vi "Read Description map.vi"(8 "error in (no error)":errorcluster, 11 "Test Tree in":refnum<class "Test Tree.lvclass">) -> (0 "error out":errorcluster, 2 "Description map":map{string, string}(c390), 3 "Test Tree out":refnum<class "Test Tree.lvclass">)   [LabVIEW 2020, in "Test Tree.lvclass"]
uses:
  Test Tree.lvclass
  Test Tree.lvclass/Test Tree.ctl
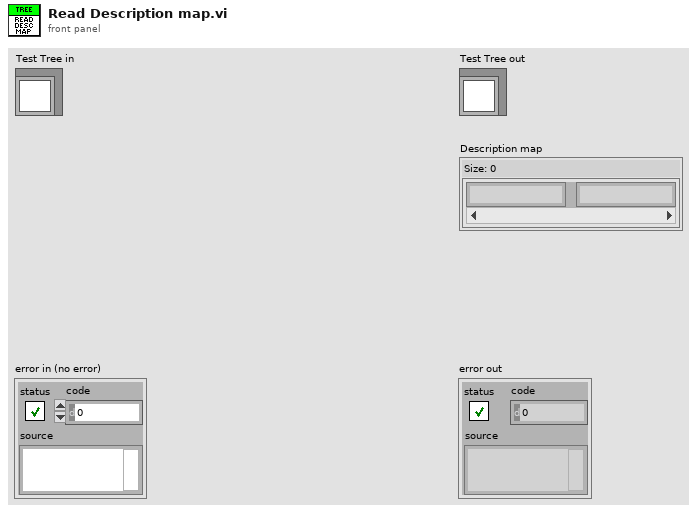
[diagram p1: front panel]
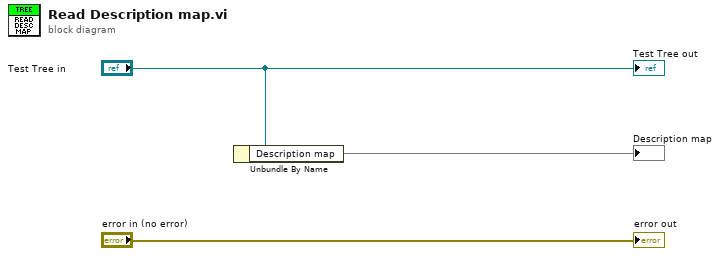
[diagram p0: block diagram]
diagram:
  n1 = Unbundle By Name("Test Tree in") -> ("Description map"=→"Description map":map{string, string})
  "error out" <- "error in (no error)"
  "Test Tree out" <- "Test Tree in"
